vi "BRig_Host__Loop_Producer__tcp_System__Data_storeFiles_v2.vi"(0 "input_arrPath_source_wExpPrefix":path[](array[path]), 1 "input_exist_sourceAny":bool[](array[boolean]), 2 "input_exist_source":bool[](array[boolean]), 3 "input_exist_source_wExpPrefix":bool[](array[boolean]), 5 "input_arrPath_source":path[](array[path]), 7 "input_arrPath_target_wExpPrefix":path[](array[path]), 9 "input_arrPath_target":path[](array[path]), 11 "input_n":i32, 12 "input_store_wExpPrefix":bool[](array[boolean]), 13 "input_storeAny":bool[](array[boolean]), 14 "input_firstPass":bool) -> (4 "output_stored_wExpPrefix":bool[](array[boolean]), 8 "output_storedAny":bool[](array[boolean]))   [LabVIEW 2014]
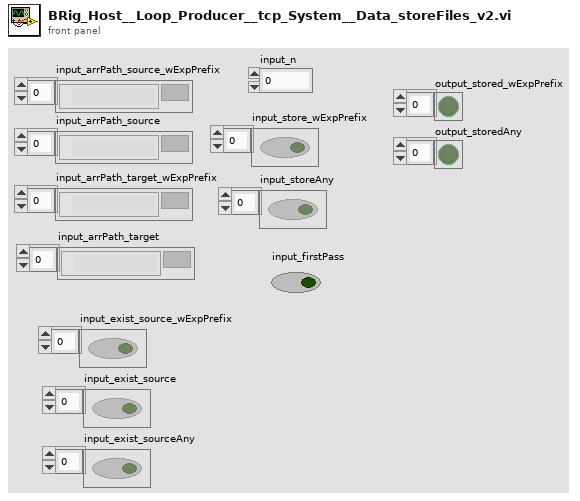
[diagram p1: front panel]
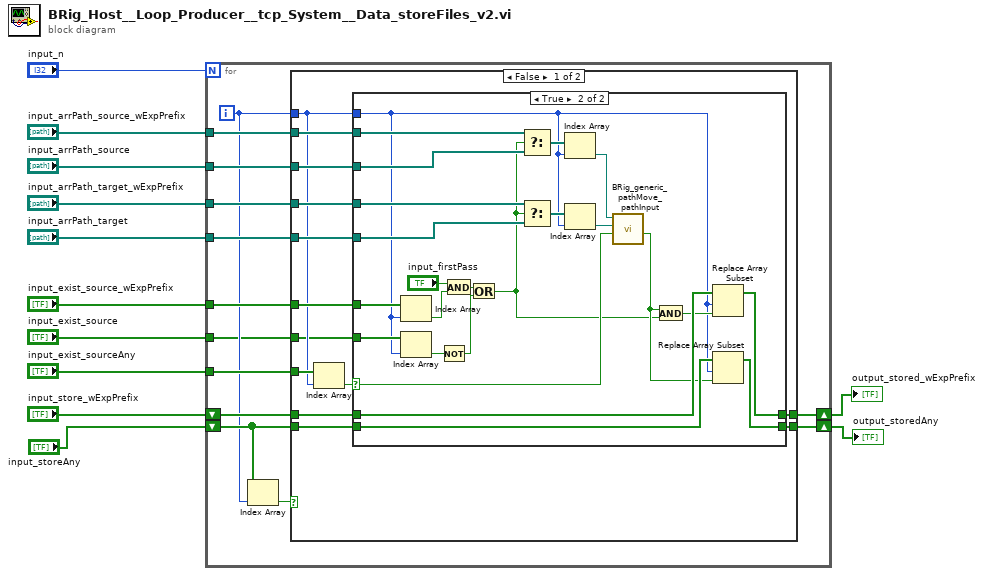
[diagram p0: block diagram]
diagram:
  n1 = for {
    N: "input_n" -> [_]
    tunnel: "input_arrPath_source" -> [w22]
    tunnel: "input_arrPath_source_wExpPrefix" -> [w23]
    tunnel: "input_arrPath_target_wExpPrefix" -> [w21]
    tunnel: "input_arrPath_target" -> [w20]
    tunnel: "input_exist_sourceAny" -> [w25]
    tunnel: "input_exist_source" -> [w13]
    tunnel: "input_exist_source_wExpPrefix" -> [w24]
    shift-right: [w18] -> w3
    shift-left: "input_store_wExpPrefix" -> [w19]
    shift-right: [w17] -> w2
    shift-left: "input_storeAny" -> [w16]
    i -> [w15]
    n2 = Index Array(array=w16, index=w15) -> (element=w14:bool)
    n3 = case shown="False" w14 {
      tunnel: w25 -> [w38 _]
      tunnel: w24 -> [w36 _]
      tunnel: w23 -> [w35 _]
      tunnel: w22 -> [w34 _]
      tunnel: w21 -> [w33 _]
      tunnel: w20 -> [w32 _]
      tunnel: w19 -> [w31 w66]
      tunnel: [w30 w66] -> w18
      tunnel: [w29 w65] -> w17
      tunnel: w16 -> [w28 w65]
      tunnel: w15 -> [w27 _]
      tunnel: w13 -> [w26 _]
      frame False {
        n4 = Index Array(array=w38, index=w27) -> (element=w37:bool)
        n5 = case shown="True" w37 {
          selector: w37 -> [_ w55]
          tunnel: w36 -> [_ w64]
          tunnel: w27 -> [_ w44]
          tunnel: w35 -> [_ w63]
          tunnel: w34 -> [_ w62]
          tunnel: w33 -> [_ w61]
          tunnel: w32 -> [_ w60]
          tunnel: w31 -> [w40 w54]
          tunnel: w28 -> [w39 w52]
          tunnel: [w40 w49] -> w30
          tunnel: [w39 w50] -> w29
          tunnel: w26 -> [_ w45]
          frame False {
          }
          frame True {
            n6 = Index Array(array=w64, index=w44) -> (element=w46:bool)
            n7 = Index Array(array=w45, index=w44) -> (element=w43:bool)
            n8 = Not(x=w43) -> (.not. x?=w42:bool)
            n9 = And(x="input_firstPass", y=w46) -> (x .and. y?=w48:bool)
            n10 = Or(x=w48, y=w42) -> (x .or. y?=w41:bool)
            n11 = Select(t=w63, s=w41, f=w62) -> (s? t:f=w59:path[])
            n12 = Select(t=w61, s=w41, f=w60) -> (s? t:f=w58:path[])
            n13 = Index Array(array=w59, index=w44) -> (element=w56:path)
            n14 = Index Array(array=w58, index=w44) -> (element=w57:path)
            n15 = call "BRig_generic_pathMove_pathInput.vi"("input_Ioverwrite"=w55, "input_filePath_target"=w57, "input_filePath_source"=w56) -> ("output_Iexist"=w51:bool)  [unwired: 6 in, 2 out]
            n16 = And(x=w51, y=w41) -> (x .and. y?=w53:bool)
            n17 = Replace Array Subset(array=w54, new element=w53, index=w44) -> (w49:bool[])
            n18 = Replace Array Subset(array=w52, new element=w51, index=w44) -> (w50:bool[])
          }
        }
      }
      frame True {
      }
    }
  }
  "output_stored_wExpPrefix" <- w3
  "output_storedAny" <- w2
